vi "LowLvCtrl_GV.vi"() -> ()   [LabVIEW 2016]
panel:
  in  "MTP Folder":path=path "c:/MotorParam"
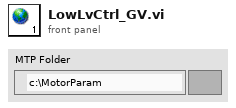
[diagram p1: front panel]
diagram:
